vi "ZK注射泵操作步.vi"(7 "是否启用通讯通知":bool, 8 "error in (no error)":errorcluster, 10 "注射泵操作步":u16, 11 "Slave ID":T1) -> (0 "error out":errorcluster)   [LabVIEW 2016, in "质控单元V4.lvlib"]
uses:
  <vilib>/Plasmionique/MB Master/MB_Master/MB_Master.lvclass
  <vilib>/Plasmionique/MB Master/MB Master.lvlib
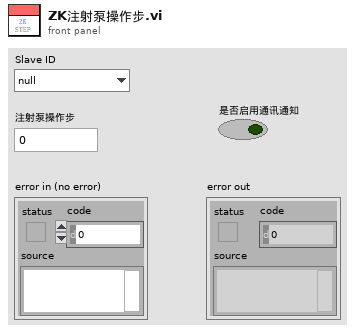
[diagram p1: front panel]
types:
  T1 = typedef "质控单元V4.lvlib/质控slave id.ctl" = enum16{"null", "氨氮", "总磷", "总氮", "CODMn", "CODCr", "氨氮总磷", "总磷总氮"}
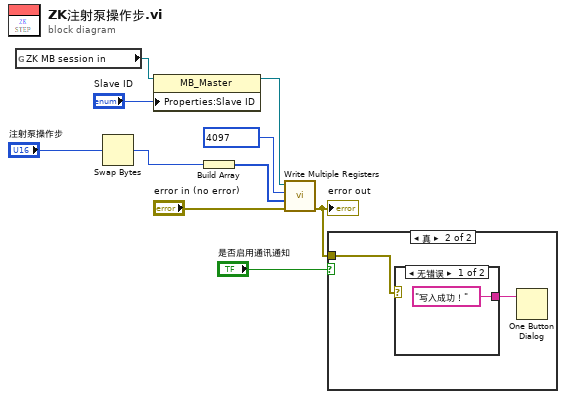
[diagram p0: block diagram]
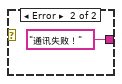
[diagram p3: hidden frame]
diagram:
  n1 = global read "ZK非断电保存全局变量.vi" "ZK MB session in"() -> (w9:refnum<class "MB_Master.lvclass">)
  n2 = Swap Bytes(anything="注射泵操作步") -> (byte swapped=w4:u16)
  n3 = property class="MB_Master"(reference=w9, "Properties:Slave ID"="Slave ID") -> (reference out=w6:refnum<class "MB_Master.lvclass">)  [unwired: 1 in, 1 out]
  n4 = Build Array(w4) -> (w3:u16[])
  n5 = call <vilib>:"Write Multiple Registers.vi"("error in (no error)"="error in (no error)", "values"=w3, "starting address"=u16 4097, "MB session in"=w6) -> ("error out"=w1:errorcluster)  [unwired: 6 in, 1 out]
  "error out" <- w1
  n6 = case shown="真" "是否启用通讯通知" {
    tunnel: w1 -> [_ w12]
    frame False {
    }
    frame True {
      n7 = case shown="无错误" w12 {
        tunnel: ["写入成功！" "通讯失败！"] -> w11
        frame No Error {
        }
        frame Error {
        }
      }
      n8 = One Button Dialog(message=w11) -> ()  [unwired: 1 in, 1 out]
    }
  }
